vi "Encode Update from Git.vi"(11 "Git update cluster":T1) -> (3 "Encoded message":string[](array[string]))   [LabVIEW 2026, in "TALOS.lvlib" / "Guardian.lvlib" / "Guardian.lvclass"]
uses:
  Guardian.lvclass
  Git Update Cluster.ctl
  TALOS.lvlib
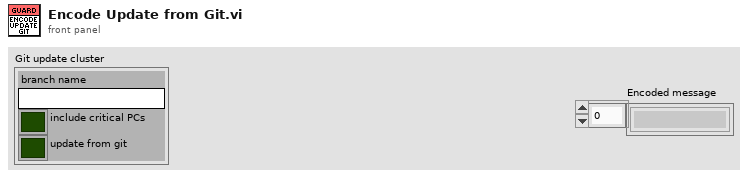
[diagram p1: front panel]
types:
  T1 = typedef "TALOS.lvlib/Guardian.lvlib/Guardian.lvclass/Git Update Cluster.ctl" = cluster{"branch name":string, "include critical PCs":bool, "update from git":bool}
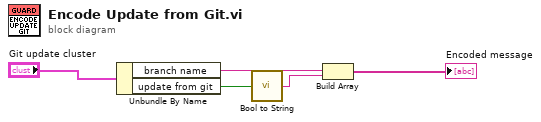
[diagram p0: block diagram]
diagram:
  n1 = Unbundle By Name("Git update cluster") -> ("branch name"=w3:string, "update from git"=w4:bool)
  n2 = call "Bool to String.vi"("Boolean"=w4) -> ("String"=w2:string)
  n3 = Build Array(w3, w2) -> (→"Encoded message":string[])
